vi "Intake Loop.vi"   [LabVIEW 2015]
uses:
  Common Code/Intake States.ctl
  Robot Global Data.vi
types:
  T1 = typedef "Intake Commands Cluster.ctl" = cluster{"Intake Commands":T2, "Intake Mode":T3, "Override IR":bool}
  T2 = typedef "Intake Commands.ctl" = enum16{"Unload", "Load", "Pull up", "Drop low", "Idle", "Lift Half"}
  T3 = typedef "Intake Mode.ctl" = enum16{"Safe", "Auto", "Manual"}
  T4 = typedef "Dashboard Control Data.ctl" = cluster{"Encoder Control":T5, "Steer PID output":cluster{"output high":dbl, "output low":dbl}, " Steer PID gains":cluster{"proportional gain (Kc)":dbl, "integral time (Ti, min)":dbl, "derivative time (Td, min)":dbl}, "Drivetrain Settings":T6, "Vision Packet":T7, "Info/Command Cluster":T8, "Ball Vision Packet":T9, "Intake Presets":T11, "Intake Encoder Control":T13, "Climb Presets":T14, "Goal Output Range":cluster{"output high":dbl, "output low":dbl}, "Shooter Presets":T15}
  T5 = typedef "Encoder Control.ctl" = cluster{"Right Tick Constant":dbl, "Left Tick Constant":dbl, "Reset?":bool, "Y Dist":cluster{"PID gains":cluster{"proportional gain (Kc)":dbl, "integral time (Ti, min)":dbl, "derivative time (Td, min)":dbl}}, "Y Stop Thresh":dbl, "Y Stop Speed":dbl}
  T6 = typedef "Drivetrain Settings.ctl" = cluster{"Gyro Tolerance":dbl, "Throttle Ramp (ms)":dbl, "Angular rate compensation":bool, "Throttle to Rate Scale":dbl, "Rate compensation gain":dbl, "Kv":dbl, "Ka":dbl, "Feed Forward P":dbl, "Feed Forward D":dbl, "Goal Vision PID gains":cluster{"proportional gain (Kc)":dbl, "integral time (Ti, min)":dbl, "derivative time (Td, min)":dbl}, "Goal Detection Window":dbl}
  T7 = typedef "Goal Vision Packet.ctl" = cluster{"Distance":dbl, "Center X":dbl, "Center Y":dbl, "Found Target?":bool}
  T8 = typedef "Ball Tracking Command Cluster.ctl" = cluster{"Distance to Ball":dbl, "Desired Angle":dbl, "Command":enum16{"Turn to Ball", "Turn to Angle", "Get Distance"}, "Pixels from Center":dbl}
  T9 = typedef "Ball Vision Packet.ctl" = cluster{"Ball Detected?":bool, "Distance to Ball":dbl, "Desired Angle":dbl, "Pixels from Center":dbl, "Tracking mode":T10}
  T10 = typedef "Tracking Mode.ctl" = enum16{"Turn to Ball", "Turn to Angle"}
  T11 = typedef "Intake Presets.ctl" = cluster{"Intake Speed":dbl, "Outake Speed":dbl, "Low Height":dbl, "Half Height":dbl, "Full Height":dbl, "Angle Speed":dbl, "Fast Angle":dbl, "Encoder Scale":dbl, "Load Height":dbl, "Output Range":T12, "Rotation Power Max/Min":dbl, "MaxCurrent":dbl, "Intake Trip Time":dbl, "Idle Height":dbl, "Max Height":dbl, "Reset Encoders?":bool, "PID gains":cluster{"proportional gain (Kc)":dbl, "integral time (Ti, min)":dbl, "derivative time (Td, min)":dbl}}
  T12 = typedef "Drivetrain Output Range.ctl" = cluster{"output high":dbl, "output low":dbl}
  T13 = typedef "IntakeEcoderControl.ctl" = cluster{"Arm Tick Constant":dbl, "Reset?":bool, "Y Dist":cluster{"PID gains":cluster{"proportional gain (Kc)":dbl, "integral time (Ti, min)":dbl, "derivative time (Td, min)":dbl}}, "Y Stop Thresh":dbl, "Y Stop Speed":dbl}
  T14 = typedef "Climb Presets.ctl" = cluster{"Pull Power":dbl, "Unpin Power":dbl, "Time to Hold":dbl}
  T15 = typedef "Shooter Presets.ctl" = cluster{"Batter Shot":T16, "Deep Middle Shot":T16, "Manual Shot":T16, "Left Ticks Per Rotation":dbl, "Right Ticks Per Rotation":dbl, "Low Bar Shot":T16, "Shooter RPM Tolerance":dbl, "IIR Filter Power":dbl, "Trigger Power":dbl, "Fire from Load Delay":i32, "Angle Pot M":dbl, "Angle Pot B":dbl, "Shooter Length":dbl, "String Pot Dist":dbl, "Angle PID gains":cluster{"proportional gain (Kc)":dbl, "integral time (Ti, min)":dbl, "derivative time (Td, min)":dbl}, "Angle Motor Output":cluster{"output high":dbl, "output low":dbl}, "Shooter Angle Tolerance":dbl, "Vision Shoot x^2":dbl, "Vision Shoot x":dbl, "Dist from Axis Cam to Pivot":dbl, "High Goal Center Height":dbl, "Feed Forward Max Accel":dbl, "Feed Forward Kv":dbl, "Backwards Trigger":dbl, "Shot Finish Delay (ms)":dbl, "Angle Max Current":dbl, "Angle Current Trip Time":dbl, "Shooter Intake Angle":dbl, "Vision Shoot c":dbl, "Reset?":bool, "Servo Release Delay":dbl, "Servo Idle Angle":i32, "Servo Hold Angle":i32, "Angle Pot x^2":dbl, "Angle Pot x":dbl, "Angle Pot c":dbl}
  T16 = typedef "Shot Presets.ctl" = cluster{"Left Wheel RPM":dbl, "Right Wheel RPM":dbl, "Angle":dbl}
  T17 = typedef "WPI_MotorControlDeviceRef.ctl" = cluster{"DeviceStatus":errorcluster, "Type":T18, "PWM":cluster{"PWM Channel":T19, "DeadBand":T20}, "CAN":cluster{"Device Number":u8, "Control Mode":T21, "Semaphore":T22, "Max Vout":dbl, "TalonSRX Control Mode":T23}, "Invert":bool}
  T18 = typedef "WPI_MotorControlType.ctl" = enum16{"PWM", "CAN", "CANTalonSRX"}
  T19 = typedef "FPGA_DIOPWMChannel.ctl" = enum8{"PWM 0", "PWM 1", "PWM 2", "PWM 3", "PWM 4", "PWM 5", "PWM 6", "PWM 7", "PWM 8", "PWM 9", "PWM MXP 0", "PWM MXP 1", "PWM MXP 2", "PWM MXP 3", "PWM MXP 4", "PWM MXP 5", "PWM MXP 6", "PWM MXP 7", "PWM MXP 8", "PWM MXP 9", "Invalid"}
  T20 = typedef "WPI_PWMDeadband.ctl" = cluster{"Name":string, "maxPositivePwm":i32, "minPositivePwm":i32, "centerPwm":i32, "maxNegativePwm":i32, "minNegativePwm":i32, "angularRange":u16}
  T21 = typedef "WPI_CANJaguar_ControlMode.ctl" = enum8{"Percent VBus", "Current", "Speed", "Position", "Voltage"}
  T22 = typedef "Semaphore RefNum" = refnum<k1>
  T23 = typedef "WPI_CANTalonSRX_APIControlMode.ctl" = enum8{"Percent VBus", "Speed", "Position", "Slave", "Unchanged / Invalid", "Voltage Compensation", "Current", "Motion Profile"}
  T24 = typedef "Intake States.ctl" = enum16{"Idle", "Set roller speed", "Move to angle"}
  T25 = typedef "Intake Status Cluster.ctl" = cluster{"Roller Power":dbl, "Angle Power":dbl, "Intake Mode":T3, "Intake States":T24, "Rollers Active?":bool, "Current Height":dbl, "Target Height":dbl, "Encoder Raw Position":dbl, "Forward Tripped?":bool, "Backward Tripped?":bool, "Override IR?":bool}
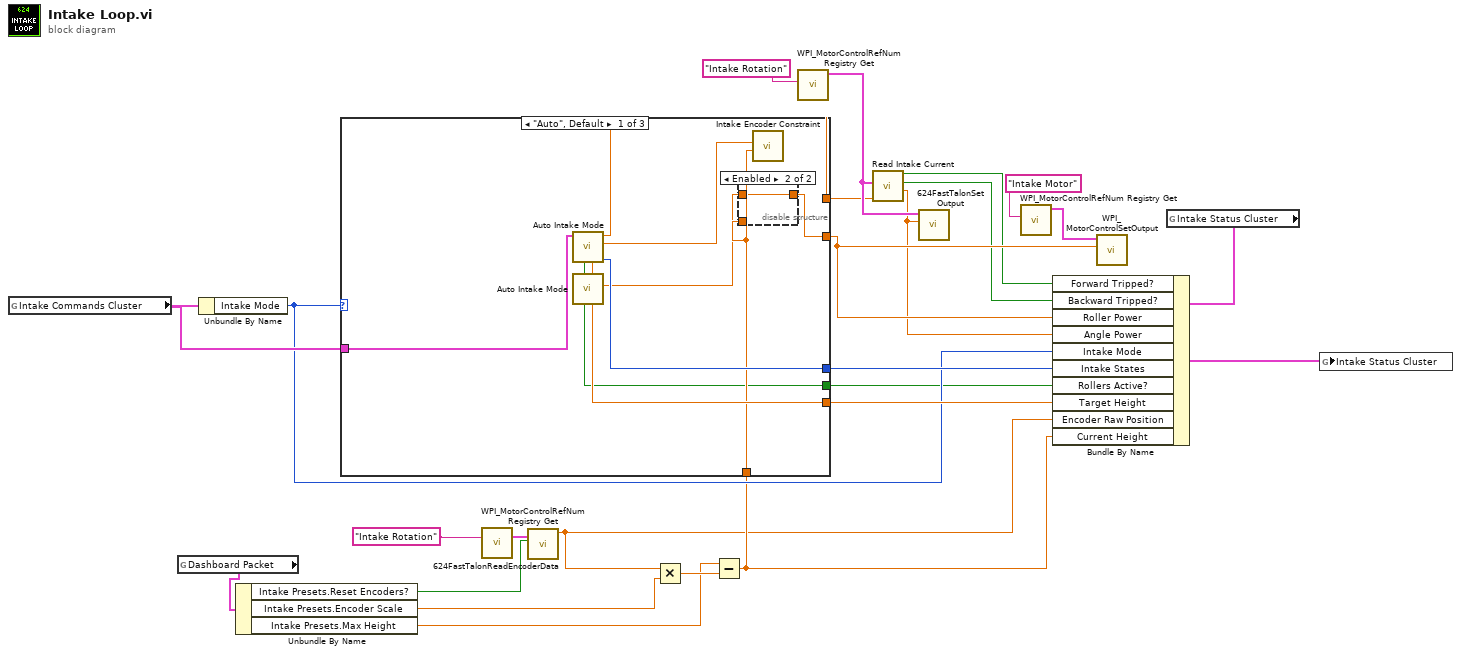
[diagram p0: block diagram]
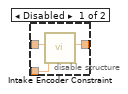
[diagram p2: hidden frame]
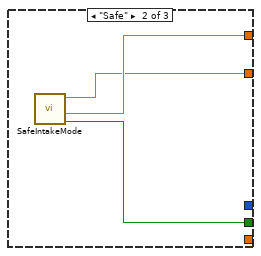
[diagram p3: hidden frame]
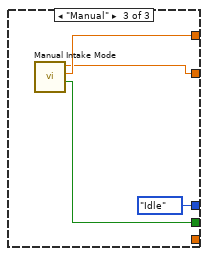
[diagram p4: hidden frame]
diagram:
  n1 = global read "Robot Global Data.vi" "Intake Commands Cluster"() -> (w25:T1)
  n2 = global read "Robot Global Data.vi" "Dashboard Packet"() -> (w2:T4)
  n3 = Unbundle By Name(w25) -> ("Intake Mode"=w17:T3)
  n4 = Unbundle By Name(w2) -> ("Intake Presets.Reset Encoders?"=w5:bool, "Intake Presets.Encoder Scale"=w4:dbl, "Intake Presets.Max Height"=w3:dbl)
  n5 = call <vilib>:"WPI_MotorControlRefNum Registry Get.vi"("refnum name"="Intake Rotation") -> ("MotorControlDevRef"=w14:T17)  [unwired: 9 in, 1 out]
  n6 = call "624FastTalonReadEncoderData.vi"("Reset?"=w5, "CAN Talon SRX Ref"=w14) -> ("Encoder Position"=w1:dbl)  [unwired: 4 in, 5 out]
  n7 = Multiply(x=w1, y=w4) -> (x*y=w6:dbl)
  n8 = Subtract(x=w3, y=w6) -> (x-y=w7:dbl)
  n9 = case shown="\"Auto\", Default" w17 {
    tunnel: w25 -> [w34 _ _]
    tunnel: [w32 w41 w44] -> w12
    tunnel: [w27 w40 w43] -> w21
    tunnel: [w30 _ Intake_States."Idle" ("Intake States")] -> w19
    tunnel: [w33 _ _] -> w18
    tunnel: w7 -> [w29 _ _]
    tunnel: [w28 w39 w42] -> w8
    frame "Auto", Default {
      n10 = call "Auto Intake Mode.vi"("Intake Commands Cluster"=w34) -> ("Intake States"=w30:T24, "Roller Power"=w31:dbl, "Angle Power"=w32:dbl, "Target Height"=w33:dbl, "Rollers Active?"=w28:bool)  [unwired: 4 in, 2 out]
      n11 = call "Auto Intake Mode.vi"() -> ("Roller Power"=w26:dbl)  [unwired: 5 in, 6 out]
      n12 = disable-structure shown="Enabled" {
        disable-tunnel: [w35 w38] -> w27
        disable-tunnel: w26 -> [w37 w38]
        disable-tunnel: w29 -> [w36 _]
        frame Disabled {
          n13 = call "Intake Encoder Constraint.vi"("Roller Power"=w37, "Encoder Position"=w36) -> ("Roller Power"=w35:dbl)  [unwired: 8 in]
        }
        frame Enabled {
        }
      }
      n14 = call "Intake Encoder Constraint.vi"("Roller Power"=w31, "Encoder Position"=w29) -> ()  [unwired: 8 in, 1 out]
    }
    frame "Safe" {
      n15 = call "SafeIntakeMode.vi"() -> ("Rollers Active?"=w39:bool, "Angle Power"=w41:dbl, "Roller Power"=w40:dbl)  [unwired: 9 in]
    }
    frame "Manual" {
      n16 = call "Manual Intake Mode.vi"() -> ("Rollers Active?"=w42:bool, "Arm Power"=w44:dbl, "Intake Power"=w43:dbl)  [unwired: 9 in]
    }
  }
  n17 = call <vilib>:"WPI_MotorControlRefNum Registry Get.vi"("refnum name"="Intake Rotation") -> ("MotorControlDevRef"=w13:T17)  [unwired: 9 in, 1 out]
  n18 = call "Read Intake Current.vi"("Proposed Power"=w12, "CAN Talon SRX Ref"=w13) -> ("Actual Power"=w11:dbl, "Reverse Trip?"=w9:bool, "Forward Trip?"=w10:bool)  [unwired: 7 in]
  n19 = call "624FastTalonSetOutput.vi"("Output"=w11, "MotorControlDevRef"=w13) -> ()  [unwired: 8 in, 2 out]
  n20 = call <vilib>:"WPI_MotorControlRefNum Registry Get.vi"("refnum name"="Intake Motor") -> ("MotorControlDevRef"=w23:T17)  [unwired: 9 in, 1 out]
  n21 = call <vilib>:"WPI_MotorControlSetOutput.vi"("Output"=w21, "MotorControlDevRef"=w23) -> ()  [unwired: 7 in, 3 out]
  n22 = global read "Robot Global Data.vi" "Intake Status Cluster"() -> (w16:T25)
  n23 = Bundle By Name(cluster=w16, "Forward Tripped?"=w10, "Backward Tripped?"=w9, "Roller Power"=w21, "Angle Power"=w11, "Intake Mode"=w17, "Intake States"=w19, "Rollers Active?"=w8, "Target Height"=w18, "Encoder Raw Position"=w1, "Current Height"=w7) -> (w20:T25)
  n24 = global write "Robot Global Data.vi" "Intake Status Cluster"(w20) -> ()
